vi "1.4.3-Drive Encoder.vi"   [LabVIEW 2011]
doc: "Encoder has part number DB-37F-SS-1000-ABCZ-72-SCS18-28\nThis translates to 1000 ticks per rotation.\nThe gear ratio is 10 teeth on the encoder sprocket to 30 teeth on the wheel sprocket.\nWheel Diameter is 15.5 inches approximately.\nWhippin out the trusty MATLAB, wheel circumferance is about 48.7 inches, and so the inches per tick is about 0.01623156 inches or 4.1228e-004 meters.\n5 mph, a reasonable speed, is 2.351 meters per second, which is 5.4214e+003 tics per second.\nif we loop every 10 ms we get updates every e-2 seconds, so we would see 54.214 each loop if we were going 5 mph. If we low pass this with n=2 we would have a speed accurate up to about 40 ms which is still plenty fast enough. Our unit for speed will be ticks per hundreth of a second. from -128 to 128 with 18 bits of resolution."
uses:
  1.0-Hindbrain Global.vi
  <vilib>/rvi/eio/common/nirviEmuTemplateMethod_errors.vi
  <vilib>/eio/EIONode/EIONode.xnode
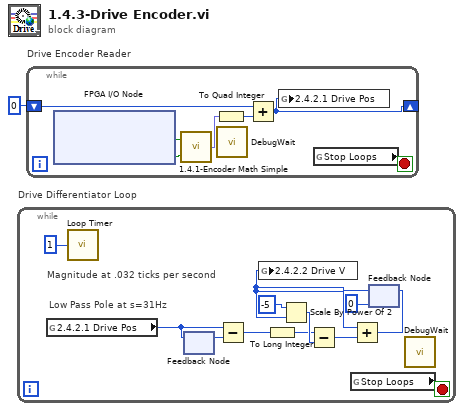
[diagram p0: block diagram]
diagram:
  n1 = while "Drive Differentiator Loop" {
    stop <- w12 stop-if-true
    # "Magnitude at .032 ticks per second"
    # "Low Pass Pole at s=31Hz"
    n2 = global read "1.0-Hindbrain Global.vi" "2.4.2.1 Drive Pos"() -> (w11:i64)
    n3 = call "Loop Timer"("Count(mSec)"=u32 1 ("Count(Ticks)")) -> ()  [unwired: 1 out]
    n4 = feedback #1() -> (w10:i64)  [unwired: 1 in]
    n5 = feedback-in #1(w11) -> ()
    n6 = Subtract(x=w11, y=w10) -> (x-y=w7:i64)
    n7 = To Long Integer(number=w7) -> (32bit integer=w3:i32)
    n8 = global read "1.0-Hindbrain Global.vi" "Stop Loops"() -> (w12:bool)
    n9 = feedback #2(0 ("2.4.2.2 Drive V")) -> (w2:i32)
    n10 = global write "1.0-Hindbrain Global.vi" "2.4.2.2 Drive V"(w2) -> ()
    n11 = Scale By Power Of 2(n=i16 -5, x=w2) -> (x*2^n=w8:i32)
    n12 = Subtract(x=w3, y=w8) -> (x-y=w6:i32)
    n13 = Add(x=w2, y=w6) -> (x+y=w5:i32)
    n14 = feedback-in #2(w5) -> ()
    n15 = call "DebugWait.vi"() -> ()  [unwired: 12 in]
  }
  n16 = while "Drive Encoder Reader" {
    shift-right: [w14] -> _
    shift-left: i64 0 ("2.4.2.1 Drive Pos") -> [w16]
    stop <- w20 stop-if-true
    n17 = xnode "FPGA I/O Node"() -> ("DriveEncoderB"=w18:bool, "DriveEncoderA"=w19:bool)  [unwired: 2 in, 2 out]
    n18 = call "1.4.1-Encoder Math Simple.vi"("B"=w19, "A"=w18) -> ("Numeric"=w17:fxp<+/-,2,2>)
    n19 = To Quad Integer(1:w17) -> (0:w15:i64)
    n20 = call "DebugWait.vi"() -> ()  [unwired: 12 in]
    n21 = Add(x=w16, y=w15) -> (x+y=w14:i64)
    n22 = global write "1.0-Hindbrain Global.vi" "2.4.2.1 Drive Pos"(w14) -> ()
    n23 = global read "1.0-Hindbrain Global.vi" "Stop Loops"() -> (w20:bool)
  }
